vi "MotorDC.vi"() -> ()   [LabVIEW 2015]
uses:
  <vilib>/imath/engines/lvmath/Plug In/Control Design/BuiltInFunctions/tf/NIMS_CD_tf(STR,Ts).vi
  <vilib>/imathl/engines/lvmath/Functions/Error Handling/Create Error.vi
  <vilib>/imath/engines/lvmath/Plug In/Control Design/BuiltInFunctions/ss/NIMS_CD_ss(A,B,C,D).vi
  <vilib>/imath/engines/lvmath2/RunTimeEngine/NodeEndStatement/NIMS_NodeEndStatement_Output.vi
  <vilib>/imath/engines/lvmath2/RunTimeEngine/ErrorHandling/NIMS_Finalize Error.vi
  <vilib>/addons/Control Design/_Utility/NI_CD_Model Viewer.lvlib
  <vilib>/addons/Control Design/_Utility/Model Viewer.llb/Model Viewer SubVI/cd_Draw Transfer Function Equation (TF).vi
  <vilib>/addons/Control Design/_Frequency Response Analysis/NI_CD_Frequency Response.lvlib
  <vilib>/addons/Control Design/_Frequency Response Analysis/Frequency Response.llb/Frequency Response subVI/cd_Bode (Transfer Function).vi
  <vilib>/addons/Control Design/_Model Construction/NI_LinSys_Model Creation.lvlib
  <vilib>/addons/Control Design/_Model Construction/Model Creation.llb/Model Creation SubVI/cd_Create State Space Model.vi
  <vilib>/addons/Control Design/_Utility/Model Viewer.llb/Model Viewer SubVI/cd_Draw State-Space Equation (SS).vi
  <vilib>/addons/Control Design/_Frequency Response Analysis/Frequency Response.llb/Frequency Response subVI/cd_Bode (State Space).vi
  <vilib>/imath/engines/lvmath/Plug In/Control Design/BuiltInFunctions/powermx/NIMS_CD_powermx(TF,N).vi
  <vilib>/imath/engines/lvmath/Plug In/Control Design/BuiltInFunctions/multmx/NIMS_CD_multmx(K,TF).vi
  <vilib>/imath/engines/lvmath/Plug In/Control Design/BuiltInFunctions/plus/NIMS_CD_plus(TF,TF).vi
  <vilib>/imath/engines/lvmath/Functions/Error Handling/MergeErrorsWrapper.vi
  <vilib>/imath/engines/lvmath/Plug In/Control Design/BuiltInFunctions/plus/NIMS_CD_plus(TF,K).vi
  <vilib>/imath/engines/lvmath/Plug In/Control Design/BuiltInFunctions/rightdivmx/NIMS_CD_rightdivmx(K,TF).vi
  <vilib>/imath/engines/lvmath/Plug In/Control Design/BuiltInFunctions/tf/NIMS_CD_tf(num,den,Ts).vi
  <vilib>/imath/engines/lvmath/Plug In/Control Design/BuiltInFunctions/tf/NIMS_CD_tf(K,Ts).vi
  <vilib>/imath/engines/lvmath2/RunTimeEngine/RowToken/NIMS_RowToken_M_CV.vi
  <vilib>/imath/engines/lvmath2/RunTimeEngine/RowToken/NIMS_RowToken_M_M.vi
  <vilib>/imath/engines/lvmath2/RunTimeEngine/ErrorHandling/NIMS_Create Error From Enums.vi
  <vilib>/addons/Control Design/_Model Interconnection/NI_CD_Model Interconnection.lvlib
  <vilib>/addons/Control Design/_Model Interconnection/Model Interconnection.llb/Model Interconnection SubVI/cd_Sensitivity Functions (SS and TF).vi
  <vilib>/addons/Control Design/_Model Conversions/NI_CD_Model Type.lvlib
  <vilib>/addons/Control Design/_Model Conversions/Model Type.llb/Model Conversion SubVI/cd_Convert State-Space to Transfer Function Model.vi
  <vilib>/imath/engines/lvmath/Plug In/Control Design/BuiltInFunctions/poleplace/NIMS_CD_poleplace(A,B,poles,STR).vi
  <vilib>/imath/engines/lvmath/Plug In/Control Design/BuiltInFunctions/rightdivmx/NIMS_CD_rightdivmx(TF,TF).vi
  <vilib>/imath/engines/lvmath/Plug In/Control Design/BuiltInFunctions/multmx/NIMS_CD_multmx(SS,TF).vi
  <vilib>/imath/engines/lvmath/Plug In/Control Design/BuiltInFunctions/feedback/NIMS_CD_feedback(SS,K,SIGN).vi
  DCMCT/Courseware/VIs/QNET Library/QNET_Drivers.llb/QNET_DCMCT_Motor_Write.vi
  DCMCT/Courseware/VIs/QNET Library/QNET_Drivers.llb/QNET_DCMCT_Speed_Current_Read.vi
  DCMCT/Courseware/VIs/QNET Library/QNET_DCMCT_Functions/DCMCT_Speed_Digital_Scopes.vi
  DCMCT/Courseware/VIs/QNET Library/QNET_DCMCT_Functions/DCMCT_Disturbance.vi
  DCMCT/Courseware/VIs/QNET Library/QNET_Signal_Generator.vi
  <vilib>/Simulation/ContinuousLinear/Implementation/NILVSim Transfer Function.llb/SIM Transfer Function (SISO).vi
  <vilib>/Simulation/Implementation/XNodeFramework/SimXNode/SimX.xnode
  <vilib>/Simulation/Utility/Implementation/SIM Time.vi
  <vilib>/Simulation/Utility/Implementation/SIM Halt.vi
  <vilib>/Simulation/SignalDisplay/Implementation/NILVSim Time Waveform.llb/SIM Time Waveform (vector).vi
  <vilib>/Simulation/Implementation/Shared/SIMSCR Execution Mode.ctl
  <vilib>/Simulation/Scripting/Companion Diagram/SimConfigNode/_simSolvers.ctl
  <vilib>/Simulation/Scripting/Companion Diagram/SimConfigNode/SimParams.ctl
  <vilib>/Simulation/Scripting/Companion Diagram/SimConfigNode/SimDog.xnode
  <vilib>/Simulation/SignalDisplay/Implementation/NILVSim Time Waveform.llb/SIM Time Waveform (scalar).vi
  <vilib>/addons/Control Design/_Model Construction/Model Typedefs.llb/CD General Elements.ctl
  <vilib>/addons/Control Design/_Model Construction/NI_LinSys_Model Typedefs.lvlib
  <vilib>/addons/Control Design/_Model Construction/Model Typedefs.llb/CD Transfer Function Model (SISO).ctl
  <vilib>/addons/Control Design/_Model Construction/Model Typedefs.llb/CD Transfer Function Model (MIMO).ctl
  <vilib>/Simulation/ContinuousLinear/Implementation/NILVSim Transfer Function.llb/SIM Transfer Function (SISO CD).vi
panel:
  in  "Stop Iteration":bool
  in  "Tab Control":T1(tab)
  out "Rm nominal":dbl
  out "Kt nominal":dbl
  out "Km nominal":dbl
  out "Jm nominal":dbl
  out "Ml nominal":dbl
  out "rl nominal":dbl
  out "L nominal":dbl
  out "Bm nominal":dbl
  out "Wp(s)":picture
  out "Bode Magnitude Nominal Plant P(s)":cluster{"W":dbl[], "Magnitude":dbl[]}[](graph)
  out "Wu(s)":picture
  out "M":dbl[][](array[numeric])
  out "P(s)":picture
  out "Inverse Wp(s)":cluster{"W":dbl[], "Magnitude":dbl[]}[](graph)
  out "Sensitivity Function":picture
  out "Comp. Sensitivity Func":picture
  out "Comp. Sens. Func":cluster{"W":dbl[], "Magnitude":dbl[]}[](graph)
  out "Speed (rad/s)":waveform(dbl)[](graph)
  in  "Stop Running":bool
  in  "Sampling Rate (Hz)":dbl=100.0 min=0.0 max=1000.0 step=25.0 format="%.1f"
  in  "Device":tag="Dev1" caption="dev"
  out "Digital Scopes":T2 {"Voltage" format="%.1f"; "Current" format="%.1f"}
  in  "Signal Generator Parameters":T3={"Amplitude"=25.0, "Frequency"=0.4, "Offset"=100.0, "Signal Type"=0, "Disturbance"=FALSE} caption="Signal Generator" {"Offset" min=0.0 max=200.0 step=5.0 format="%.1f"; "Frequency" min=0.0 step=0.1 format="%.2f"; "Amplitude" min=0.0 max=100.0 step=5.0 format="%.1f"}
  out "Voltage (V)":waveform(dbl)(graph)
  out "Sensitivity Func":cluster{"W":dbl[], "Magnitude":dbl[]}[](graph)
  out "Close Loop using PID":cluster{"W":dbl[], "Magnitude":dbl[]}[](graph)
  out "Digital Scopes Hinf":T2 {"Voltage" format="%.1f"; "Current" format="%.1f"}
  in  "Sampling Rate Hinf(Hz)":dbl=100.0 min=0.0 max=1000.0 step=25.0 format="%.1f"
  in  "Signal Generator Parameters 2":T3={"Amplitude"=25.0, "Frequency"=0.4, "Offset"=100.0, "Signal Type"=0, "Disturbance"=FALSE} caption="Signal Generator" {"Offset" min=0.0 max=200.0 step=5.0 format="%.1f"; "Frequency" min=0.0 step=0.1 format="%.2f"; "Amplitude" min=0.0 max=100.0 step=5.0 format="%.1f"}
  out "Speed Hinf (rad/s)":waveform(dbl)[](graph) caption="Speed (rad/s)"
  in  "Device Hinf":tag="Dev1" caption="dev"
  out "Voltage (V) Hinf":waveform(dbl)(graph)
  out "Sensitivity Function Hinf":picture
  out "Comp. Sensitivity Func Hinf":picture
  out "Close Loop using Hinf":cluster{"W":dbl[], "Magnitude":dbl[]}[](graph)
  out "Sensitivity Func Hinf":cluster{"W":dbl[], "Magnitude":dbl[]}[](graph)
  out "Comp. Sens. Func Hinf":cluster{"W":dbl[], "Magnitude":dbl[]}[](graph)
  # "Robust Control for DC Motor Speed Control using H_infinity"
  # "By : Fajri, Alif, Aulia, Khansa and Ovi"
  # "Supervisor : Prof. Dr. Ir. Bambang Riyanto Trilakso"
  # "System Interconnection G_dcm"
  # "rad/s"
  # "A"
  # "V"
  # "rad/s"
  # "Hz"
  # "rad/s"
  # "rad/s"
  # "A"
  # "V"
  # "rad/s"
  # "Hz"
  # "rad/s"
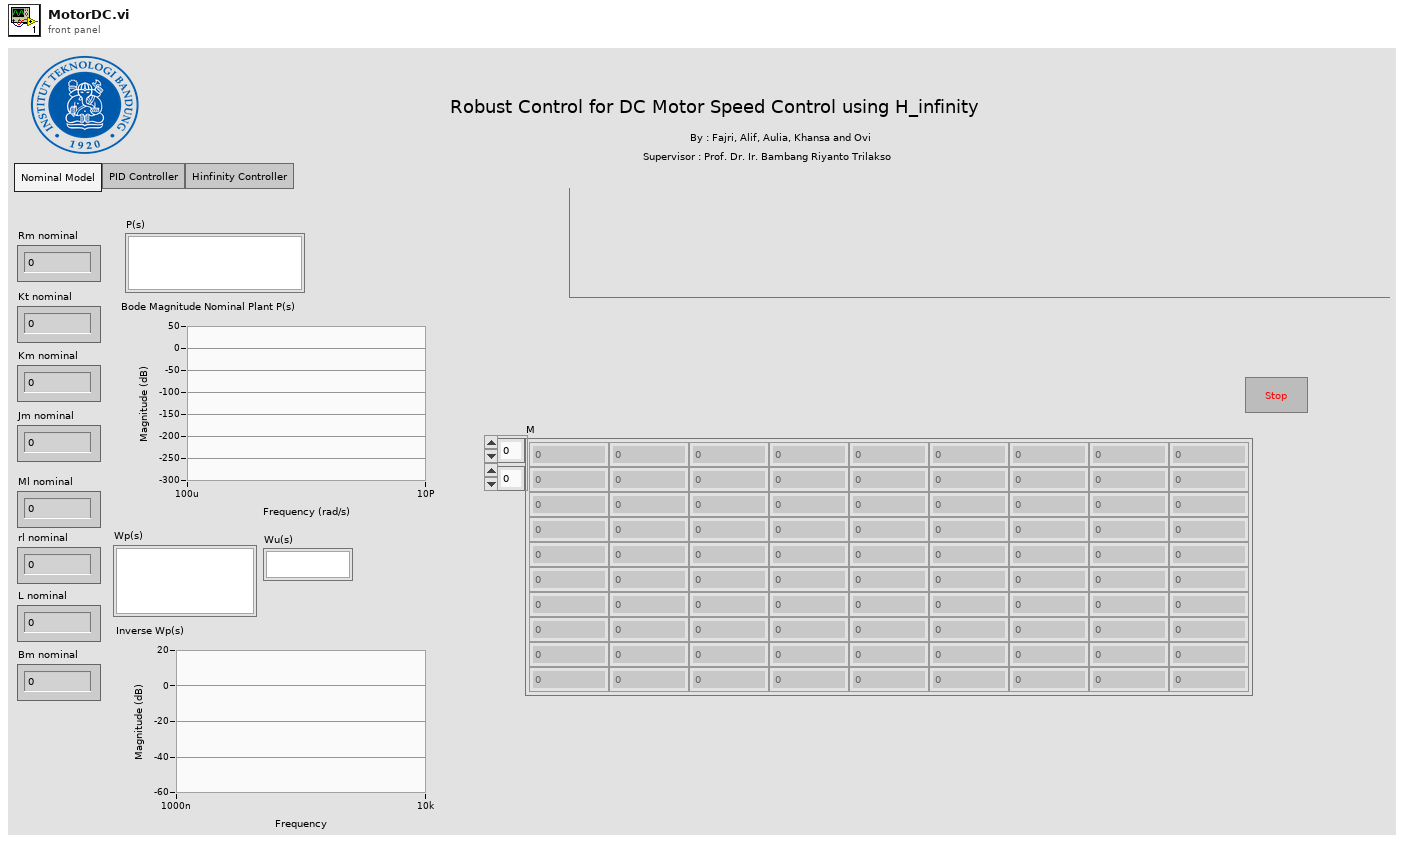
[diagram p1: front panel]
types:
  T1 = enum32{"Nominal Model", "PID Controller", "Hinfinity Controller"}
  T2 = cluster{"Current":dbl, "Voltage":dbl, "Speed":dbl}
  T3 = cluster{"Amplitude":dbl, "Frequency":dbl, "Offset":dbl, "Signal Type":u16, "Disturbance":bool}
  T4 = typedef "SimParams.ctl" = cluster{"Initial Time (s)":dbl, "Final Time (s)":dbl, "Step Size (s)":dbl, "ODE Solver":T5, "Minimum Step Size (s)":dbl, "Maximum Step Size (s)":dbl, "Relative Tolerance":dbl, "Absolute Tolerance":dbl, "Software Timing":bool, "Initial Step Size (s)":dbl, "Automatic Fixed Step Size?":bool, "Automatic Discrete Step Size?":bool, "Discrete Step Size (s)":dbl, "Calculate using Time Step":bool, "Solver Wired?":bool, "Prev.Frm.Expected End":u64, "Prev.Frm.Actual End":u64, "Prev.Frm.Finished Late?":bool, "Prev.Iter.Expected End":u64, "Prev.Iter.Actual End":u64, "Prev.Iter.Finished Late?":bool, "Expected Iteration Start":u64, "Actual Iteration Start":u64, "Expected Frame Start":u64, "Actual Frame Start":u64, "Source Name":string, "Name":string, "Period":i64, "Deadline":i64, "Offset":i64, "Start":i64, "Priority":i32, "Timeout":i32, "Processor":i32, "Mode":enum32{"No Change", "Process missed periods, maintain original phase", "Discard missed periods, maintain original phase", "Process missed periods, ignore original phase", "Discard missed periods, ignore original phase"}, "Wakeup reason":enum32{"Normal", "Aborted", "Asynchronous wakeup", "Timing source error", "Timed loop error", "Timeout"}, "Error":errorcluster, "Source Type":string, "Secondary Source Type":string, "Global End Time":u64, "Global Start Time":u64, "Full Solver Reset":bool, "Execution Mode":T6, "Nan/Inf Check":bool, "Custom Solver Library":string, "Solver Is Variable":bool, "custom solver name":string, "Signal Collection Decimation":u32}
  T5 = typedef "_simSolvers.ctl" = enum16{"Runge-Kutta 1 (Euler)", "Runge-Kutta 2", "Runge-Kutta 3", "Runge-Kutta 4", "Runge-Kutta 23 (variable)", "Runge-Kutta 45 (variable)", "BDF (variable)", "Adams-Moulton (variable)", "Rosenbrock (variable)", "Discrete States Only", "SDIRK 4 (variable)", "Radau 5 (variable)", "Radau 9 (variable)", "Radau 13 (variable)", "Radau [Variable Order] (variable)", "Gear's Method (variable)", "Linearizer", "State Query", "Trim Eval", "Custom Solver"}
  T6 = typedef "SIMSCR Execution Mode.ctl" = enum16{"Simulate to Completion", "Single Time-Step Simulation (Fixed Step Only)"}
  T7 = typedef "NI_LinSys_Model Typedefs.lvlib/CD Transfer Function Model (MIMO).ctl" = cluster{"properties":T8, "transfer function(s)":T9[][]}
  T8 = typedef "NI_LinSys_Model Typedefs.lvlib/CD General Elements.ctl" = cluster{"Model name":string, "Input names":string[], "Output names":string[], "Input Delays":dbl[], "Output Delays":dbl[], "Sampling Time":dbl, "Notes":string}
  T9 = typedef "NI_LinSys_Model Typedefs.lvlib/CD Transfer Function Model (SISO).ctl" = cluster{"Numerator":dbl[], "Denominator":dbl[], "delay":dbl}
  T10 = typedef "NI_LinSys_Model Typedefs.lvlib/CD State Space Model (MIMO).ctl" = cluster{"properties":T8, "A":dbl[][], "B":dbl[][], "C":dbl[][], "D":dbl[][], "StateNames":string[], "Transport Delay":dbl[][]}
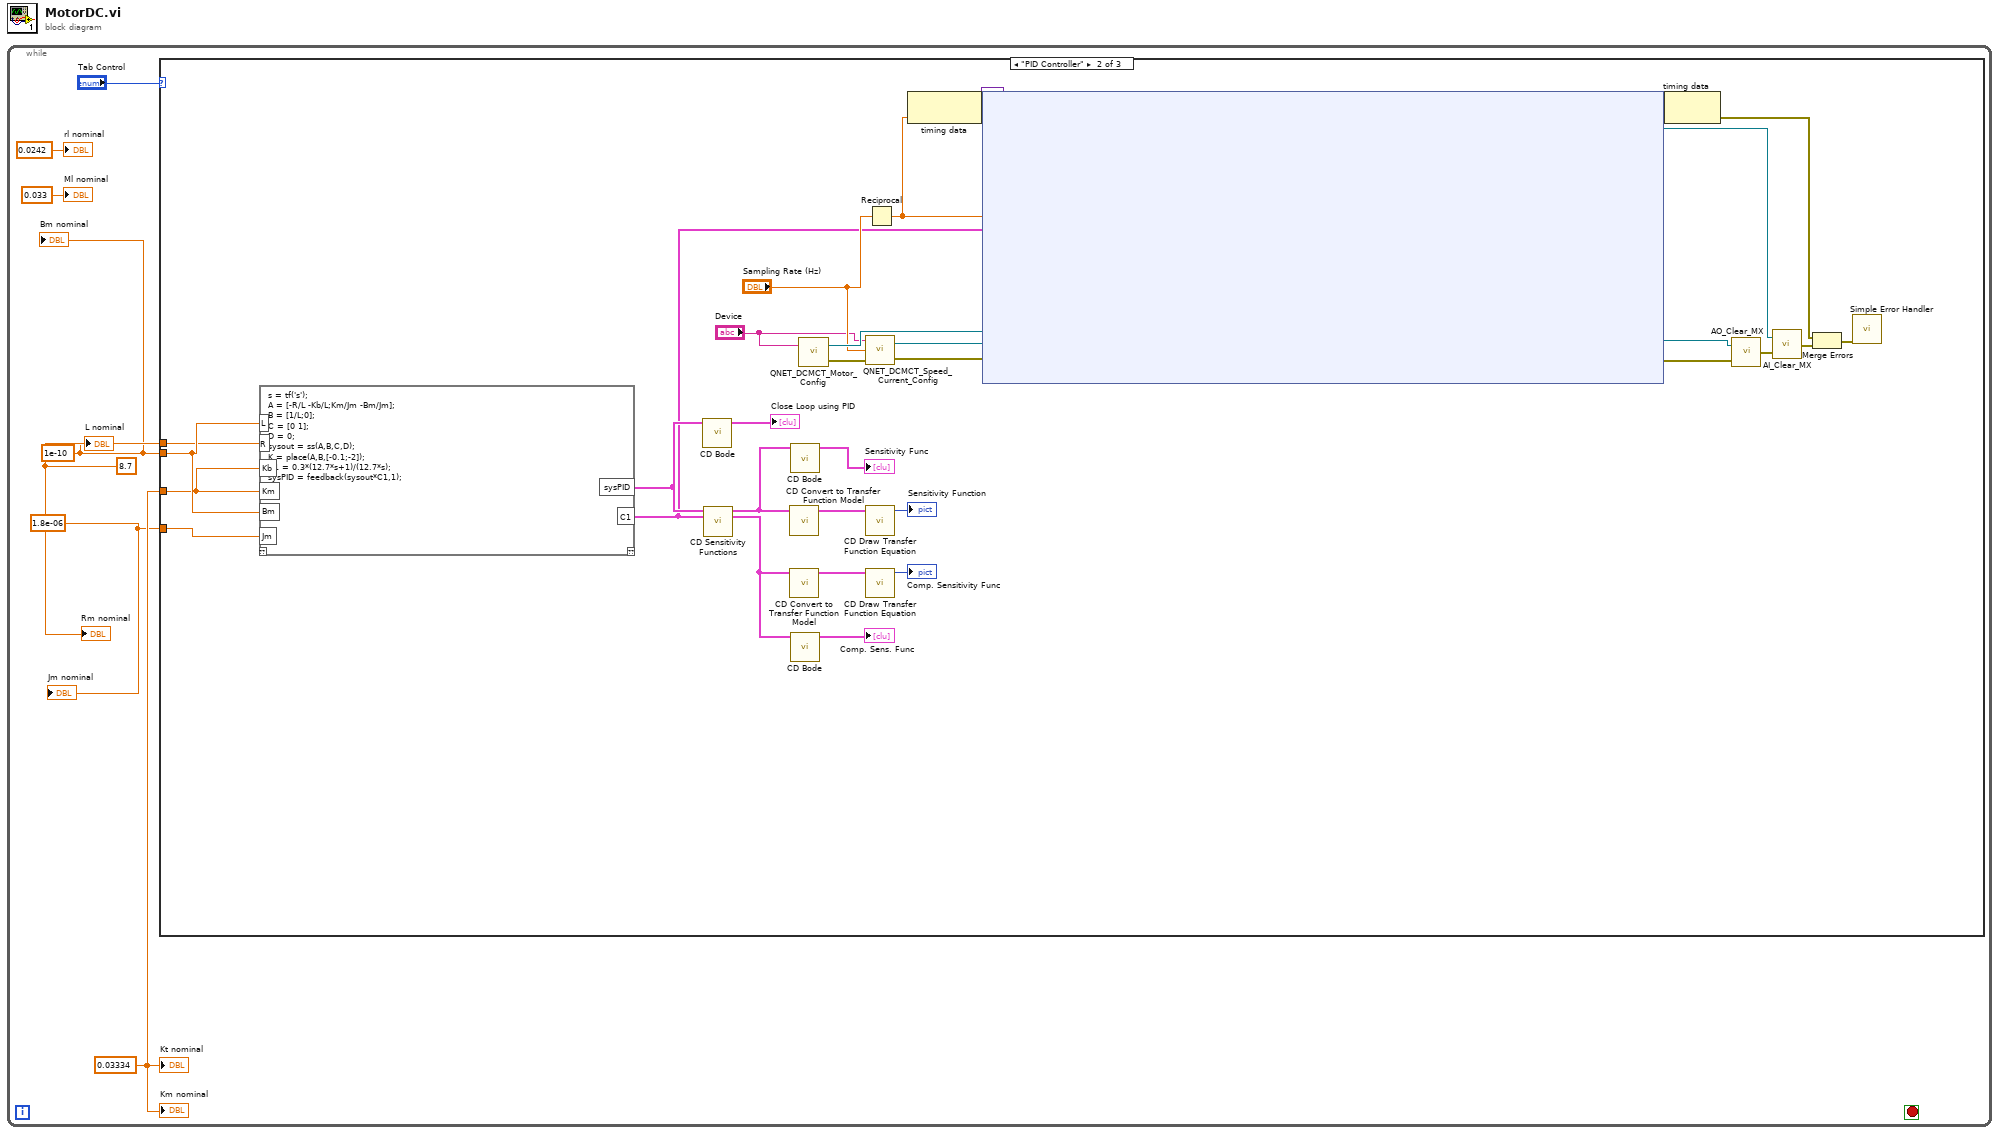
[diagram p0: block diagram]
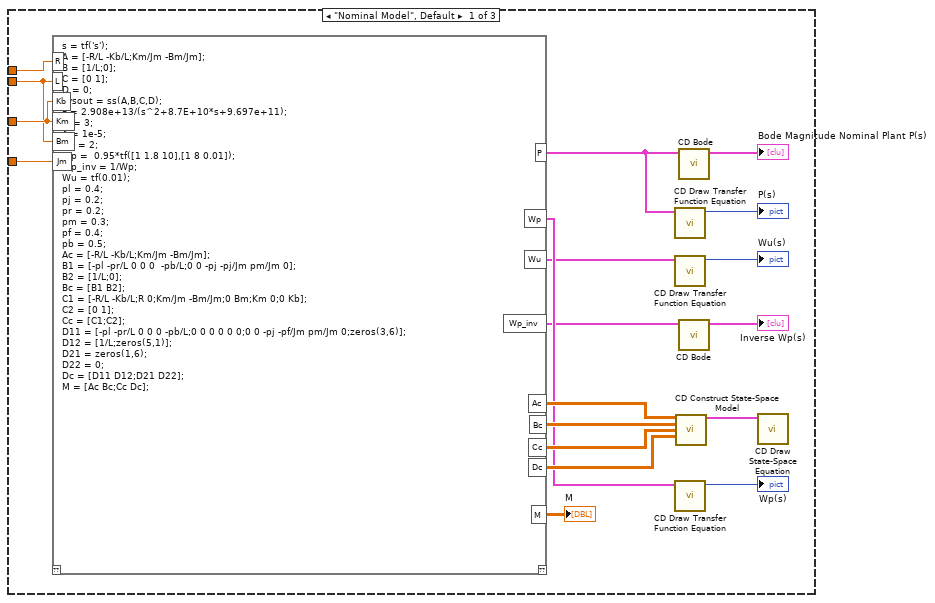
[diagram p2: hidden frame]
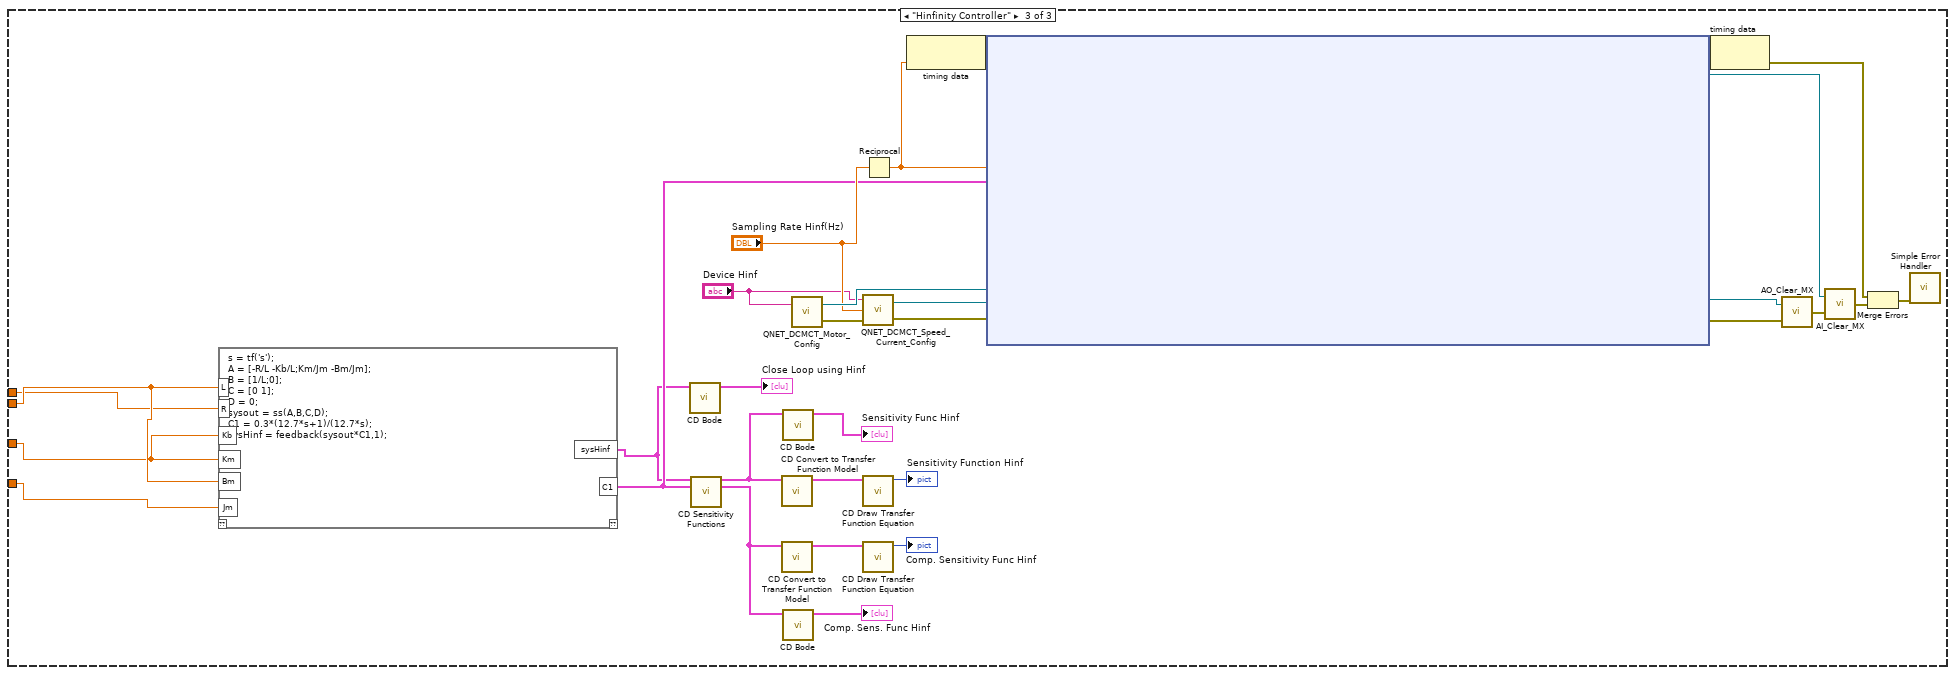
[diagram p3: hidden frame]
diagram:
  n1 = while {
    stop <- _ stop-if-true
    w4 = 1e-10 ("L nominal")
    w2 = 1.8e-06 ("Jm nominal")
    w3 = 0.03334 ("Kt nominal")
    w5 = 8.7 ("Rm nominal")
    n2 = case shown="\"PID Controller\"" "Tab Control" {
      tunnel: w5 -> [w26 w532 w754]
      tunnel: w4 -> [w24 w533 w757]
      tunnel: w3 -> [w25 w531 w755]
      tunnel: w2 -> [w23 w530 w756]
      frame "Nominal Model", Default {
        n3 = mathscript code="s = tf('s');\nA = [-R/L -Kb/L;Km/Jm -Bm/Jm];\nB = [1/L;0];\nC = [0 1];\nD = 0;\nsysout = ss(A,B,C,D);\nP = 2.908e+13/(s^2+8.7E+10*s+9.697e+11);\nM = 3;\nA = 1e-5;\nwb = 2;\nWp =  0.95*tf([1 1.8 10],[1 8 0.01]);\nWp_inv = 1/Wp;\nWu = tf(0.01);\npl = 0.4;\npj = 0.2;\npr = 0.2;\npm = 0.3;\npf = 0.4;\npb = 0.5;\nAc = [-R/L -Kb/L;Km/Jm -Bm/Jm];\nB1 = [-pl -pr/L 0 0 0  -pb/L;0 0 -pj -pj/Jm pm/Jm 0];\nB2 = [1/L;0];\nBc = [B1 B2];\nC1 = [-R/L -Kb/L;R 0;Km/Jm -Bm/Jm;0 Bm;Km 0;0 Kb];\nC2 = [0 1];\nCc = [C1;C2];\nD11 = [-pl -pr/L 0 0 0 -pb/L;0 0 0 0 0 0;0 0 -pj -pf/Jm pm/Jm 0;zeros(3,6)];\nD12 = [1/L;zeros(5,1)];\nD21 = zeros(1,6);\nD22 = 0;\nDc = [D11 D12;D21 D22];\nM = [Ac Bc;Cc Dc];"("R"=w26, "L"=w24, "Kb"=w25, "Km"=w25, "Bm"=w24, "Jm"=w23) -> ("P"=w9:T7, "Ac"=w18:dbl[][], "Bc"=w17:dbl[][], "Cc"=w16:dbl[][], "Dc"=w15:dbl[][], "Wp"=w13:T7, "Wu"=w12:T7, "Wp_inv"=w11:T7, "M"=→"M":dbl[][])  [unwired: 1 in, 1 out]
        n4 = call-poly <vilib>:"CD Draw Transfer Function Equation.vi"("Transfer Function Model"=w9) -> ("Equation"=→"P(s)":picture)  [unwired: 8 in, 2 out]
        n5 = call-poly <vilib>:"CD Draw Transfer Function Equation.vi"("Transfer Function Model"=w12) -> ("Equation"=→"Wu(s)":picture)  [unwired: 8 in, 2 out]
        n6 = call-poly <vilib>:"CD Draw Transfer Function Equation.vi"("Transfer Function Model"=w13) -> ("Equation"=→"Wp(s)":picture)  [unwired: 8 in, 2 out]
        n7 = call-poly <vilib>:"CD Construct State-Space Model.vi"("A"=w18, "B"=w17, "C"=w16, "D"=w15) -> ("State-Space Model"=w14:T10)  [unwired: 10 in, 1 out]
        n8 = call-poly <vilib>:"CD Bode.vi"("Transfer Function Model"=w9) -> ("Bode Magnitude"=→"Bode Magnitude Nominal Plant P(s)":cluster{"W":dbl[], "Magnitude":dbl[]}[])  [unwired: 6 in, 4 out]
        n9 = call-poly <vilib>:"CD Bode.vi"("Transfer Function Model"=w11) -> ("Bode Magnitude"=→"Inverse Wp(s)":cluster{"W":dbl[], "Magnitude":dbl[]}[])  [unwired: 6 in, 4 out]
        n10 = call-poly <vilib>:"CD Draw State-Space Equation.vi"("State-Space Model"=w14) -> ()  [unwired: 8 in, 3 out]
      }
      frame "PID Controller" {
        n11 = mathscript code="s = tf('s');\nA = [-R/L -Kb/L;Km/Jm -Bm/Jm];\nB = [1/L;0];\nC = [0 1];\nD = 0;\nsysout = ss(A,B,C,D);\nK = place(A,B,[-0.1;-2]);\nC1 = 0.3*(12.7*s+1)/(12.7*s);\nsysPID = feedback(sysout*C1,1);"("L"=w533, "R"=w532, "Kb"=w531, "Km"=w531, "Bm"=w533, "Jm"=w530) -> ("sysPID"=w528:T10, "C1"=w503:T7)  [unwired: 1 in, 1 out]
        n12 = call-poly <vilib>:"CD Bode.vi"("State-Space Model"=w528) -> ("Bode Magnitude"=→"Close Loop using PID":cluster{"W":dbl[], "Magnitude":dbl[]}[])  [unwired: 6 in, 4 out]
        n13 = call-poly <vilib>:"CD Sensitivity Functions.vi"("Plant Model (P)"=w528, "Controller Model (C)"=w503) -> ("Sensitivity (S)"=w523:T10, "Complementary Sensitivity (T)"=w520:T10)  [unwired: 7 in, 5 out]
        n14 = call-poly <vilib>:"CD Convert to Transfer Function Model.vi"("State-Space Model"=w523) -> ("Transfer Function Model"=w527:T7)  [unwired: 9 in, 1 out]
        n15 = call-poly <vilib>:"CD Convert to Transfer Function Model.vi"("State-Space Model"=w520) -> ("Transfer Function Model"=w524:T7)  [unwired: 9 in, 1 out]
        n16 = call-poly <vilib>:"CD Bode.vi"("State-Space Model"=w523) -> ("Bode Magnitude"=→"Sensitivity Func":cluster{"W":dbl[], "Magnitude":dbl[]}[])  [unwired: 6 in, 4 out]
        n17 = call-poly <vilib>:"CD Bode.vi"("State-Space Model"=w520) -> ("Bode Magnitude"=→"Comp. Sens. Func":cluster{"W":dbl[], "Magnitude":dbl[]}[])  [unwired: 6 in, 4 out]
        n18 = call "QNET_DCMCT_Motor_Config.vi"("dev"="Device") -> ("error out"=w511:errorcluster, "task out"=w512:refnum<k21>)  [unwired: 1 in]
        n19 = call "QNET_DCMCT_Speed_Current_Config.vi"("error in"=w511, "sampling rate (Hz)"="Sampling Rate (Hz)", "dev"="Device") -> ("error out"=w514:errorcluster, "task out"=w513:refnum<k21>)
        n20 = call-poly <vilib>:"CD Draw Transfer Function Equation.vi"("Transfer Function Model"=w527) -> ("Equation"=→"Sensitivity Function":picture)  [unwired: 8 in, 2 out]
        n21 = call-poly <vilib>:"CD Draw Transfer Function Equation.vi"("Transfer Function Model"=w524) -> ("Equation"=→"Comp. Sensitivity Func":picture)  [unwired: 8 in, 2 out]
        n22 = Reciprocal(x="Sampling Rate (Hz)") -> (1/x=w507:dbl)
        n23 = node-c288(w507) -> (w519:variant)
        n24 = node-c254 ("Simulation Loop")(w519, w514, w513, w512, w507, w503) -> (w518:variant, w517:errorcluster, w516:refnum<k21>, w515:refnum<k21>)
        n25 = node-c288(w518) -> (w506:errorcluster)
        n26 = call "AO_Clear_MX.vi"("Error in"=w517, "Task in"=w515) -> ("Error out"=w510:errorcluster)
        n27 = call "AI_Clear_MX.vi"("Error in"=w510, "Task in"=w516) -> ("Error out"=w505:errorcluster)
        n28 = Merge Errors(w506, w505) -> (w504:errorcluster)
        n29 = call <vilib>:"Simple Error Handler.vi"("error in (no error)"=w504) -> ()  [unwired: 1 in, 8 out]
      }
      frame "Hinfinity Controller" {
        n30 = mathscript code="s = tf('s');\nA = [-R/L -Kb/L;Km/Jm -Bm/Jm];\nB = [1/L;0];\nC = [0 1];\nD = 0;\nsysout = ss(A,B,C,D);\nC1 = 0.3*(12.7*s+1)/(12.7*s);\nsysHinf = feedback(sysout*C1,1);"("L"=w757, "R"=w754, "Kb"=w755, "Km"=w755, "Bm"=w757, "Jm"=w756) -> ("C1"=w758:T7, "sysHinf"=w753:T10)  [unwired: 1 in, 1 out]
        n31 = call-poly <vilib>:"CD Bode.vi"("State-Space Model"=w753) -> ("Bode Magnitude"=→"Close Loop using Hinf":cluster{"W":dbl[], "Magnitude":dbl[]}[])  [unwired: 6 in, 4 out]
        n32 = call-poly <vilib>:"CD Sensitivity Functions.vi"("Plant Model (P)"=w753, "Controller Model (C)"=w758) -> ("Sensitivity (S)"=w776:T10, "Complementary Sensitivity (T)"=w773:T10)  [unwired: 7 in, 5 out]
        n33 = call-poly <vilib>:"CD Convert to Transfer Function Model.vi"("State-Space Model"=w776) -> ("Transfer Function Model"=w780:T7)  [unwired: 9 in, 1 out]
        n34 = call-poly <vilib>:"CD Convert to Transfer Function Model.vi"("State-Space Model"=w773) -> ("Transfer Function Model"=w777:T7)  [unwired: 9 in, 1 out]
        n35 = call-poly <vilib>:"CD Bode.vi"("State-Space Model"=w776) -> ("Bode Magnitude"=→"Sensitivity Func Hinf":cluster{"W":dbl[], "Magnitude":dbl[]}[])  [unwired: 6 in, 4 out]
        n36 = call-poly <vilib>:"CD Bode.vi"("State-Space Model"=w773) -> ("Bode Magnitude"=→"Comp. Sens. Func Hinf":cluster{"W":dbl[], "Magnitude":dbl[]}[])  [unwired: 6 in, 4 out]
        n37 = call "QNET_DCMCT_Motor_Config.vi"("dev"="Device Hinf") -> ("error out"=w766:errorcluster, "task out"=w767:refnum<k21>)  [unwired: 1 in]
        n38 = call "QNET_DCMCT_Speed_Current_Config.vi"("error in"=w766, "sampling rate (Hz)"="Sampling Rate Hinf(Hz)", "dev"="Device Hinf") -> ("error out"=w769:errorcluster, "task out"=w768:refnum<k21>)
        n39 = call-poly <vilib>:"CD Draw Transfer Function Equation.vi"("Transfer Function Model"=w780) -> ("Equation"=→"Sensitivity Function Hinf":picture)  [unwired: 8 in, 2 out]
        n40 = call-poly <vilib>:"CD Draw Transfer Function Equation.vi"("Transfer Function Model"=w777) -> ("Equation"=→"Comp. Sensitivity Func Hinf":picture)  [unwired: 8 in, 2 out]
        n41 = Reciprocal(x="Sampling Rate Hinf(Hz)") -> (1/x=w762:dbl)
        n42 = node-c288(w762) -> (w783:variant)
        n43 = node-c254 ("Simulation Loop 2")(w783, w769, w768, w767, w762, w758) -> (w782:variant, w772:errorcluster, w771:refnum<k21>, w770:refnum<k21>)
        n44 = node-c288(w782) -> (w761:errorcluster)
        n45 = call "AO_Clear_MX.vi"("Error in"=w772, "Task in"=w770) -> ("Error out"=w765:errorcluster)
        n46 = call "AI_Clear_MX.vi"("Error in"=w765, "Task in"=w771) -> ("Error out"=w760:errorcluster)
        n47 = Merge Errors(w761, w760) -> (w759:errorcluster)
        n48 = call <vilib>:"Simple Error Handler.vi"("error in (no error)"=w759) -> ()  [unwired: 1 in, 8 out]
      }
    }
    "Rm nominal" <- w5
    "Kt nominal" <- w3
    "Km nominal" <- w3
    "Jm nominal" <- w2
    "Ml nominal" <- 0.033 ("Ml nominal")
    "rl nominal" <- 0.0242 ("rl nominal")
    "L nominal" <- w4
    "Bm nominal" <- w4
  }
